vi "Record Button Off.vi"(8 "error in (no error)":errorcluster, 11 "Main Window in":refnum<class "Main Window.lvclass">) -> (0 "error out":errorcluster, 3 "Main Window out":refnum<class "Main Window.lvclass">)   [LabVIEW 2015, in "Main Window.lvlib" / "Main Window.lvclass"]
uses:
  Main Window.lvclass
  <vilib>/event_ctls.llb/usereventprio.ctl
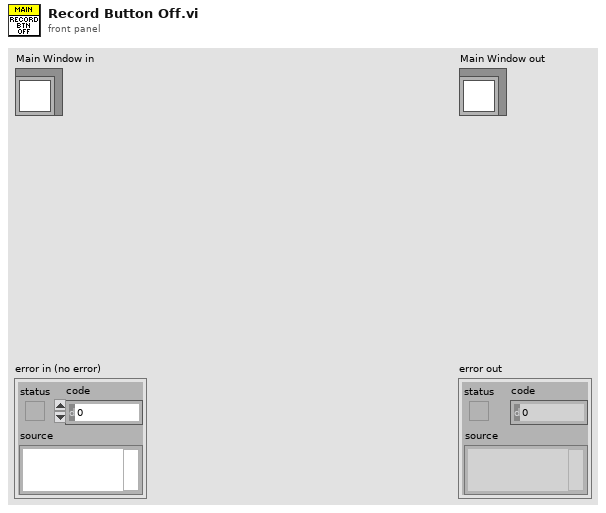
[diagram p1: front panel]
types:
  T1 = typedef "usereventprio.ctl" = enum32{"high priority", "normal priority"}
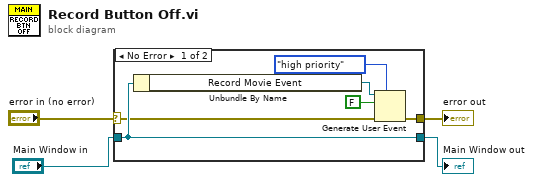
[diagram p0: block diagram]
diagram:
  n1 = case shown="No Error" "error in (no error)" {
    selector: "error in (no error)" -> [w7 w12]
    tunnel: [w6 w12] -> w3
    tunnel: [w10 w11] -> w1
    tunnel: "Main Window in" -> [w10 w11]
    frame No Error {
      n2 = Unbundle By Name(w10) -> ("Record Movie Event"=w9:refnum<user-event>)
      n3 = Generate User Event(priority (normal)=usereventprio."high priority", user event=w9, event data cluster=FALSE ("event data"), error in=w7) -> (error out=w6:errorcluster)  [unwired: 1 out]
    }
    frame Error {
    }
  }
  "error out" <- w3
  "Main Window out" <- w1
